vi "Get Current Sheet Name.vi"(8 "error in (no error)":errorcluster, 11 "MS-Excel in":refnum<class "MS-Excel.lvclass">) -> (0 "error out":errorcluster, 2 "Active Sheet Name":string, 3 "MS-Excel out":refnum<class "MS-Excel.lvclass">)   [LabVIEW 2017, in "LabVIEW NPOI.lvlib" / "MS-Excel.lvclass"]
doc: "Returns the name, in <b>Active Sheet Name</b>, of the active worksheet of the associated workbook to the <b>Document</b>."
uses:
  MS-Excel.lvclass
  C:/Users/Neo/Desktop/Dev_Tools_BR/LabVIEW_NPOI/lib/NPOI 2.1.1/NPOI.dll
  lib/NPOI 2.1.1/NPOI.dll
  Get Current Sheet.vi
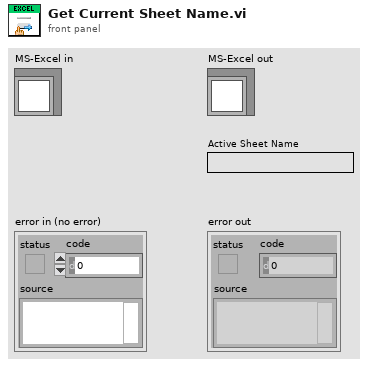
[diagram p1: front panel]
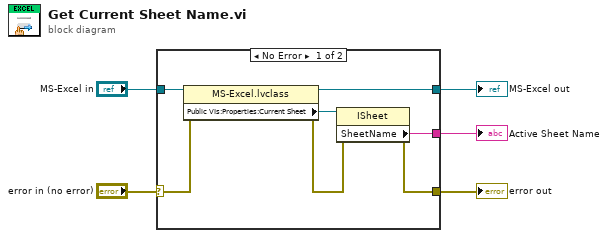
[diagram p0: block diagram]
diagram:
  n1 = case shown="No Error" "error in (no error)" {
    selector: "error in (no error)" -> [w7 w14]
    tunnel: [w11 w14] -> w4
    tunnel: [w9 w13] -> w2
    tunnel: "MS-Excel in" -> [w10 w13]
    tunnel: [w12 _] -> w1
    frame No Error {
      n2 = property class="MS-Excel.lvclass"(reference=w10, error in=w7) -> (reference out=w9:refnum<class "MS-Excel.lvclass">, error out=w6:errorcluster, "Public VIs:Properties:Current Sheet"=w8:refnum<k24>)
      n3 = property class="ISheet"(reference=w8, error in=w6) -> (error out=w11:errorcluster, "SheetName"=w12:string)  [unwired: 1 out]
    }
    frame Error {
    }
  }
  "error out" <- w4
  "MS-Excel out" <- w2
  "Active Sheet Name" <- w1
